vi "Write Mode.vi"(8 "Error In":errorcluster, 10 "Mode":T1, 11 "Session In":refnum<class "Session.lvclass">) -> (0 "Error Out":errorcluster, 3 "Sesssion Out":refnum<class "Session.lvclass">)   [LabVIEW 2017, in "LabSSH2.lvlib" / "Session.lvclass"]
uses:
  Session.lvclass
  Typedefs/Modes.ctl
  Session.lvclass/Session.ctl
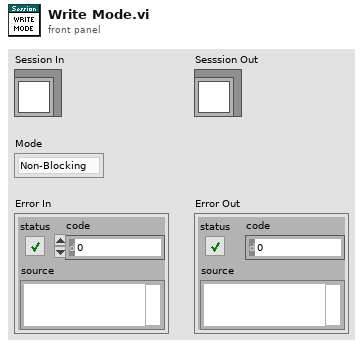
[diagram p1: front panel]
types:
  T1 = typedef "LabSSH2.lvlib/Session.lvclass/Modes.ctl" = enum16{"Non-Blocking", "Blocking"}
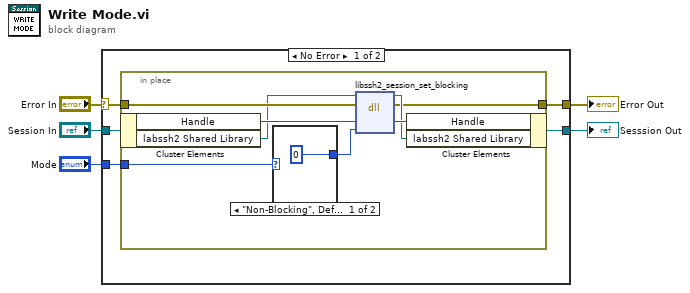
[diagram p0: block diagram]
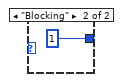
[diagram p2: hidden frame]
diagram:
  n1 = case shown="No Error" "Error In" {
    selector: "Error In" -> [w9 w22]
    tunnel: [w10 w22] -> w4
    tunnel: "Session In" -> [w8 w21]
    tunnel: [w7 w21] -> w2
    tunnel: "Mode" -> [w6 _]
    frame No Error {
      n2 = in-place {
        in-place-border: [w13] -> w10
        in-place-border: w9 -> [w18]
        in-place-border: w6 -> [w12]
        n3 = in-place-cluster #1(w8) -> ("Handle"=w17:u64, "labssh2 Shared Library"=w15:path)
        n4 = case shown="\"Non-Blocking\", Default" w12 {
          tunnel: [0 1] -> w11
          frame "Non-Blocking", Default {
          }
          frame "Blocking" {
          }
        }
        n5 = dll-call lib="D:/Users/cfield/Code/Field R&D Services/SSH/LabSSH2/LabVIEW/trunk/src/LabSSH2/Private/labssh2.*" fn="libssh2_session_set_blocking"(path in=w15, error in=w18, "session"=w17, "blocking"=w11) -> (path out=w14:path, error out=w13:errorcluster, "session"=w16:u64)  [unwired: 3 in]
        n6 = in-place-cluster #1("Handle"=w16, "labssh2 Shared Library"=w14) -> (w7:refnum<class "Session.lvclass">)
      }
    }
    frame Error {
    }
  }
  "Sesssion Out" <- w2
  "Error Out" <- w4
